vi "Data compensation.vi"(3 "Input ambient":dbl[](array[numeric]), 4 "Index":i32, 5 "Input probe":dbl[](array[numeric])) -> (0 "Output ambient":dbl, 1 "Output probe":dbl, 2 "Output probe array":dbl[](array[numeric]))   [LabVIEW 2016]
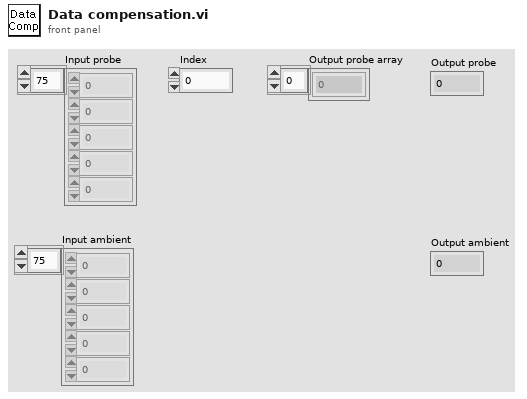
[diagram p1: front panel]
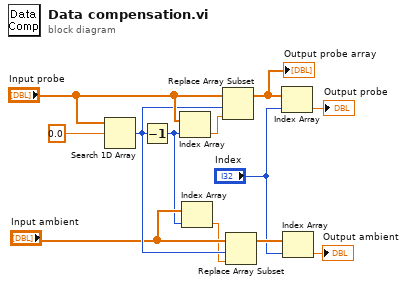
[diagram p0: block diagram]
diagram:
  n1 = Search 1D Array(1D array="Input probe", element=0.0 ("원소")) -> (index of element=w7:i32)  [unwired: 1 in]
  n2 = Decrement(x=w7) -> (x-1=w5:i32)
  n3 = Index Array(array="Input probe", index=w5) -> (element=w11:dbl)
  n4 = Index Array(array="Input ambient", index=w5) -> (element=w4:dbl)
  n5 = Replace Array Subset(array="Input probe", new element=w11, index=w7) -> (w10:dbl[])
  "Output probe array" <- w10
  n6 = Replace Array Subset(array="Input ambient", new element=w4, index=w7) -> (w3:dbl[])
  n7 = Index Array(array=w10, index="Index") -> (element=→"Output probe":dbl)
  n8 = Index Array(array=w3, index="Index") -> (element=→"Output ambient":dbl)
